vi "Anders_AnalyzeUDP_IRIS_V1_optimized.vi"(10 "Input UDP packet array":i32[][](array[numeric])=array703x1377[968031 elements]) -> (0 "Valid":bool[](array[boolean]), 2 "All good 2":bool, 3 "Return Description":T2(array[cluster]))   [LabVIEW 2018]
panel:
  out "unsigned 8bit integer":u8[](array[numeric])
  in  "Tab Control":T1(tab)
  out "Number of UDP arrays":i32
  out "All good":bool
  out "Ray sequence":u8=12
  out "Returns":u8
  out "Final size":i32=1336
  out "time stamp, ns":u32=459884670
  out "Detector":i32
  out "Line number 2":i32=146
  out "Azimuth(rad)":dbl=0.5140380859375
  out "Elevation(rad)":dbl=-0.232177734375
  out "Checkpoint":bool
  out "Returns OK":bool
  out "RESERVED3=239":bool
  out "Number of rays":u8=53
  out "found rays":i32=53
  out "# completed UDP arrays":i32
  out "size(s)":i32=42322
  # "340-400\n260-280\n97"
  # "1. Wall at 14m\n2. Dual pole= Site A+B crosstalk\n3. Edge spray is range walk"
  # "Analyze UDP IRIS V1"
  # "Ray header (for every ray)"
  # "Returns"
  # "Lidar Packet header"
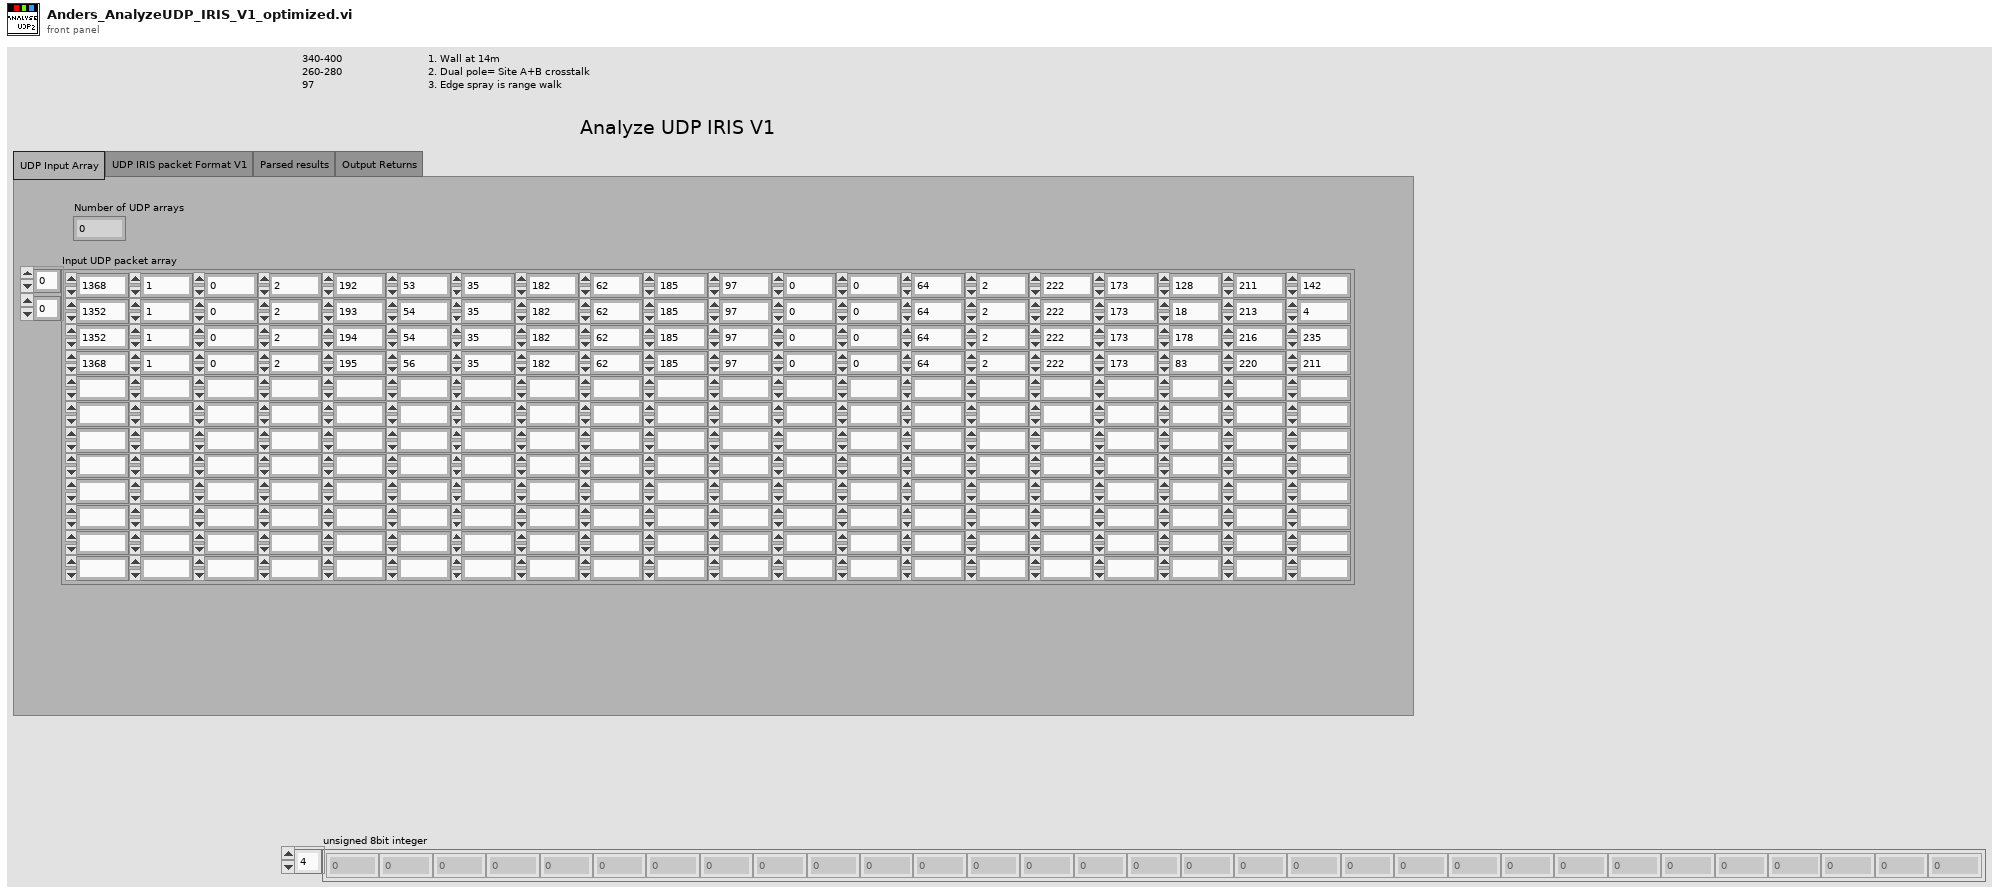
[diagram p1: front panel]
types:
  T1 = enum32{"UDP Input Array", "UDP IRIS packet Format V1", "Parsed results", "Output Returns"}
  T2 = cluster{"Azimuth":dbl, "Elevation":dbl, "Timestamp,ns":u32, "Detector":i32, "Line number":u16, "Range":ext, "Probability":ext, "Reflectance":ext, "Return":ext}[]
  T3 = cluster{dbl, dbl, "u32":u32, i32, u16, ext, ext, ext, i32}
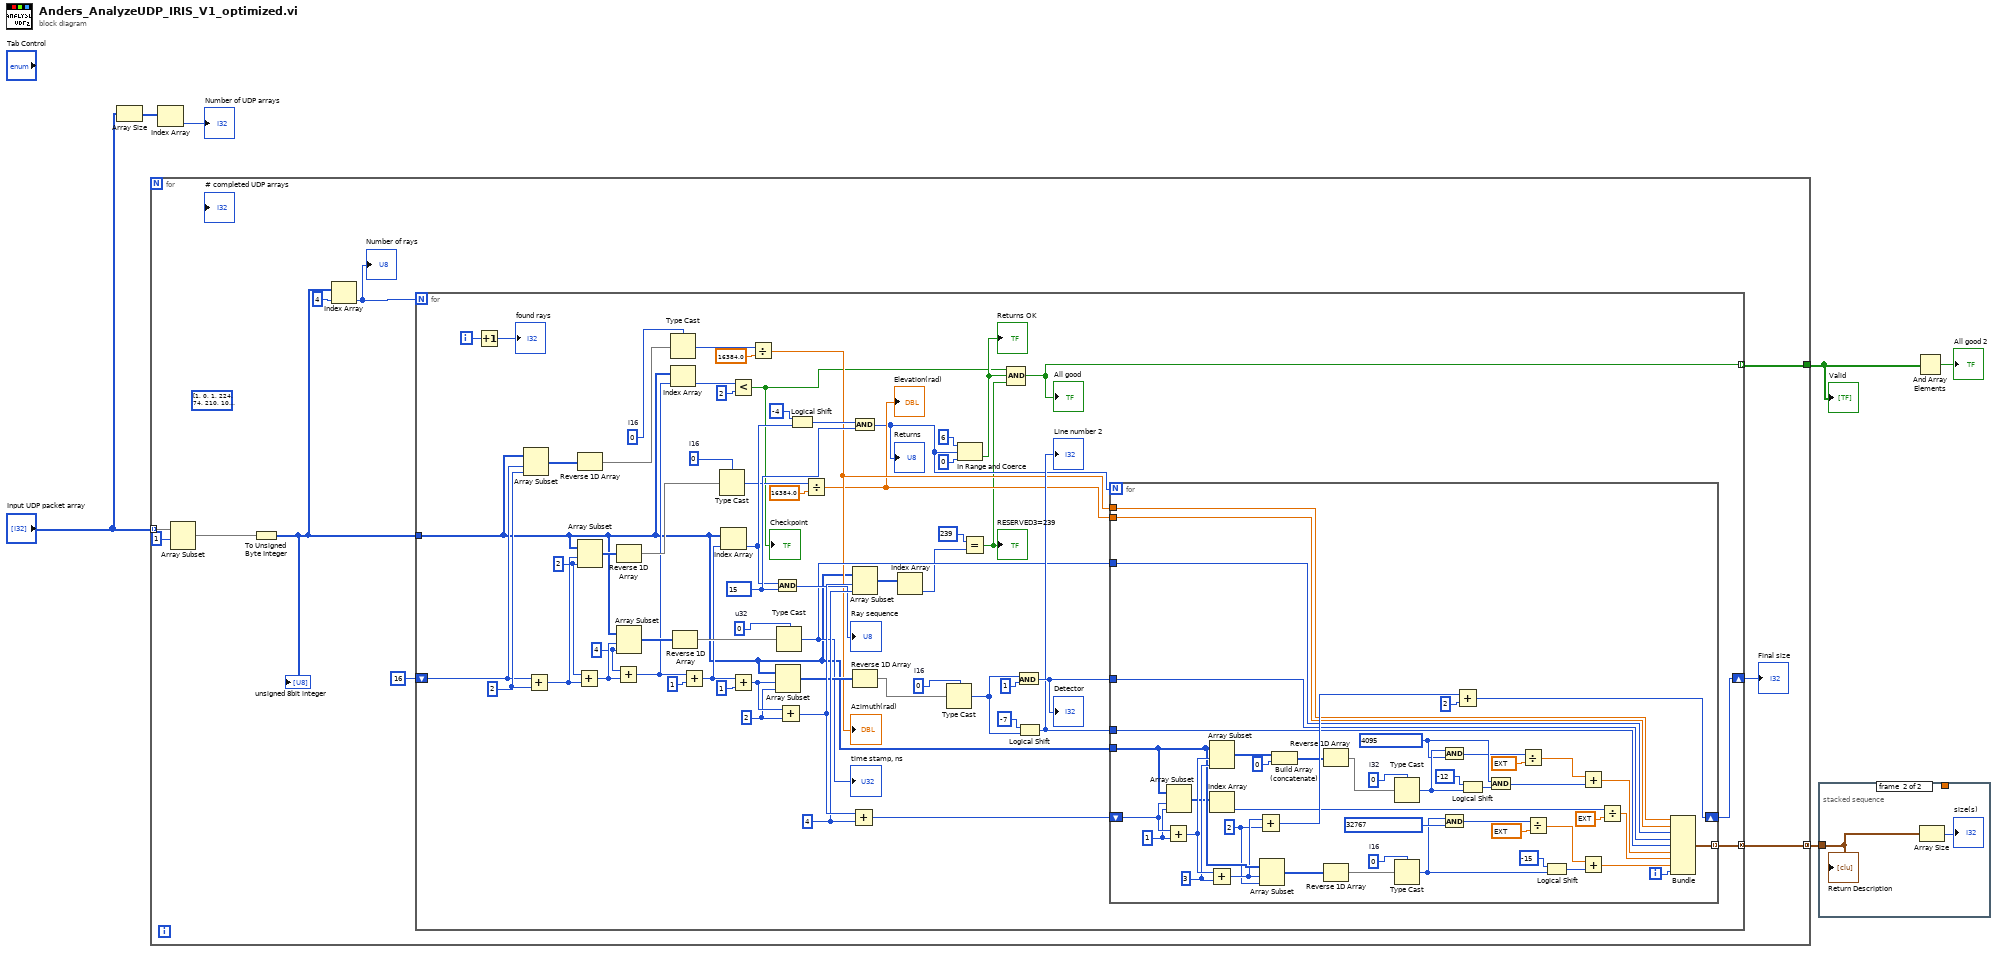
[diagram p0: block diagram]
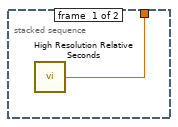
[diagram p2: hidden frame]
diagram:
  n1 = Array Size(array="Input UDP packet array") -> (size(s)=w6:i32[])
  n2 = for {
    tunnel: [w16] -> w3 mode=concatenating
    tunnel: [w15] -> w2
    tunnel: "Input UDP packet array" -> [w14] mode=indexing
    (unwired) u8[] [1, 0, 1, 224, 74, 210, 101, 1, 0, 0, 0, 0, 64, 2, 222, 173, 90, 70, 182, 0, 139, 134, 224, 18, 0, 10, 130, 50, 239, 190, 173, 222, 127, 68, 27, 0, 139, 134, 224, 18, 0, 11, 131, 50, 239, 190, 173, 222, 125, 70, 181, 0, 191, 142, 224, 18, 0, 12, 130, 50, 239, 190, 173, 222, 162, 68, 26, 0, 191, 142, 224, 18, 0, 13, 131, 50, 239, 190, 173, 222, 159, 70, 181, 0, 213, 150, 224, 18, 0, 14, 130, 50, 239, 190, 173, 222, 196, 68, 26, 0, 213, 150, 224, 18, 0, 15, 131, 50, 239, 190, 173, 222, 194, 70, 180, 0, 10, 159, 224, 18, 0, 0, 130, 50, 239, 190, 173, 222, 230, 68, 25, 0, 10, 159, 224, 18, 0, 1, 131, 50, 239, 190, 173, 222, 228, 70, 180, 0, 32, 167, 224, 18, 0, 2, 130, 50, 239, 190, 173, 222, 9, 69, 25, 0, 32, 167, 224, 18, 0, 3, 131, 50, 239, 190, 173, 222, 6, 71, 179, 0, 84, 175, 224, 18, 0, 4, 130, 50, 239, 190, 173, 222, 43, 69, 25, 0, 84, 175, 224, 18, 0, 5, 131, 50, 239, 190, 173, 222, 41, 71, 179, 0, 136, 183, 224, 18, 0, 6, 130, 50, 239, 190, 173, 222, 78, 69, 24, 0, 136, 183, 224, 18, 0, 7, 131, 50, 239, 190, 173, 222, 75, 71, 179, 0, 158, 191, 224, 18, 0, 8, 130, 50, 239, 190, 173, 222, 112, 69, 24, 0, 158, 191, 224, 18, 0, 9, 131, 50, 239, 190, 173, 222, 109, 71, 178, 0, 210, 199, 224, 18, 0, 10, 130, 50, 239, 190, 173, 222, 146, 69, 23, 0, 210, 199, 224, 18, 0, 11, 131, 50, 239, 190, 173, 222, 144, 71, 178, 0, 232, 207, 224, 18, 0, 12, 130, 50, 239, 190, 173, 222, 181, 69, 23, 0, 232, 207, 224, 18, 0, 13, 131, 50, 239, 190, 173, 222, 178, 71, 177, 0, 28, 216, 224, 18, 0, 14, 130, 50, 239, 190, 173, 222, 215, 69, 23, 0, 28, 216, 224, 18, 0, 15, 131, 50, 239, 190, 173, 222, 212, 71, 177, 0, 50, 224, 224, 18, 0, 0, 130, 50, 239, 190, 173, 222, 249, 69, 22, 0, 50, 224, 224, 18, 0, 1, 131, 50, 239, 190, 173, 222, 247, 71, 176, 0, 102, 232, 224, 18, 0, 2, 130, 50, 239, 190, 173, 222, 28, 70, 22, 0, 102, 232, 224, 18, 0, 3, 131, 50, 239, 190, 173, 222, 25, 72, 176, 0, 124, 240, 224, 18, 0, 4, 130, 50, 239, 190, 173, 222, 62, 70, 21, 0, 124, 240, 224, 18, 0, 5, 131, 50, 239, 190, 173, 222, 60, 72, 176, 0, 176, 248, 224, 18, 0, 6, 130, 50, 239, 190, 173, 222, 96, 70, 21, 0, 176, 248, 224, 18, 0, 7, 131, 50, 239, 190, 173, 222, 94, 72, 175, 0, 228, 0, 225, 18, 0, 8, 130, 50, 239, 190, 173, 222, 131, 70, 20, 0, 228, 0, 225, 18, 0, 9, 131, 50, 239, 190, 173, 222, 128, 72, 175, 0, 251, 8, 225, 18, 0, 10, 130, 50, 239, 190, 173, 222, 165, 70, 20, 0, 251, 8, 225, 18, 0, 11, 131, 50, 239, 190, 173, 222, 163, 72, 174, 0, 47, 17, 225, 18, 0, 12, 130, 50, 239, 190, 173, 222, 200, 70, 20, 0, 47, 17, 225, 18, 0, 13, 131, 50, 239, 190, 173, 222, 197, 72, 174, 0, 69, 25, 225, 18, 0, 14, 130, 50, 239, 190, 173, 222, 234, 70, 19, 0, 69, 25, 225, 18, 0, 15, 131, 50, 239, 190, 173, 222, 232, 72, 174, 0, 121, 33, 225, 18, 0, 0, 130, 50, 239, 190, 173, 222, 12, 71, 19, 0, 121, 33, 225, 18, 0, 1, 131, 50, 239, 190, 173, 222, 10, 73, 173, 0, 143, 41, 225, 18, 0, 2, 130, 50, 239, 190, 173, 222, 47, 71, 18, 0, 143, 41, 225, 18, 0, 3, 131, 50, 239, 190, 173, 222, 44, 73, 173, 0, 195, 49, 225, 18, 0, 4, 130, 50, 239, 190, 173, 222, 81, 71, 18, 0, 195, 49, 225, 18, 0, 5, 131, 50, 239, 190, 173, 222, 79, 73, 172, 0, 217, 57, 225, 18, 0, 6, 130, 50, 239, 190, 173, 222, 116, 71, 18, 0, 217, 57, 225, 18, 0, 7, 131, 50, 239, 190, 173, 222, 113, 73, 172, 0, 13, 66, 225, 18, 0, 8, 130, 50, 239, 190, 173, 222, 150, 71, 17, 0, 13, 66, 225, 18, 0, 9, 131, 50, 239, 190, 173, 222, 10, 193, 204, 0, 249, 138, 240, 18, 0, 10, 4, 51, 239, 190, 173, 222, 47, 191, 38, 0, 249, 138, 240, 18, 0, 11, 5, 51, 239, 190, 173, 222, 45, 193, 204, 0, 15, 147, 240, 18, 0, 12, 4, 51, 239, 190, 173, 222, 82, 191, 38, 0, 15, 147, 240, 18, 0, 29, 5, 51, 239, 190, 173, 222, 63, 48, 0, 0, 96, 35, 8, 0, 79, 193, 205, 0, 67, 155, 240, 18, 0, 14, 4, 51, 239, 190, 173, 222, 116, 191, 39, 0, 67, 155, 240, 18, 0, 31, 5, 51, 239, 190, 173, 222, 63, 192, 0, 0, 184, 35, 8, 0, 114, 193, 205, 0, 119, 163, 240, 18, 0, 0, 4, 51, 239, 190, 173, 222, 150, 191, 39, 0, 119, 163, 240, 18, 0, 1, 5, 51, 239, 190, 173, 222, 148, 193, 205, 0, 141, 171, 240, 18, 0, 2, 4, 51, 239, 190, 173, 222, 185, 191, 39, 0, 141, 171, 240, 18, 0, 19, 5, 51, 239, 190, 173, 222, 63, 48, 0, 0, 8, 34, 8, 0, 182, 193, 206, 0, 194, 179, 240, 18, 0, 20, 4, 51, 239, 190, 173, 222, 255, 140, 24, 0, 160, 13, 0, 0, 219, 191, 40, 0, 194, 179, 240, 18, 0, 5, 5, 51, 239, 190, 173, 222, 217, 193, 206, 0, 216, 187, 240, 18, 0, 6, 4, 51, 239, 190, 173, 222, 254, 191, 40, 0, 216, 187, 240, 18, 0, 23, 5, 51, 239, 190, 173, 222, 63, 192, 0, 0, 224, 40, 8, 0, 251, 193, 207, 0, 12, 196, 240, 18, 0, 8, 4, 51, 239, 190, 173, 222, 32, 192, 41, 0, 12, 196, 240, 18, 0, 25, 5, 51, 239, 190, 173, 222, 63, 192, 0, 0, 32, 37, 8, 0, 29, 194, 207, 0, 34, 204, 240, 18, 0, 26, 4, 51, 239, 190, 173, 222, 255, 11, 26, 0, 160, 5, 0, 0, 66, 192, 41, 0, 34, 204, 240, 18, 0, 27, 5, 51, 239, 190, 173, 222, 63, 192, 0, 0, 104, 37, 8, 0, 64, 194, 207, 0, 86, 212, 240, 18, 0, 28, 4, 51, 239, 190, 173, 222, 255, 251, 26, 0, 224, 2, 0, 0, 101, 192, 41, 0, 86, 212, 240, 18, 0, 29, 5, 51, 239, 190, 173, 222, 63, 192, 0, 0, 136, 40, 8, 0, 98, 194, 208, 0, 108, 220, 240, 18, 0, 30, 4, 51, 239, 190, 173, 222, 255, 11, 26, 0, 144, 4, 0, 0, 135, 192, 42, 0, 108, 220, 240, 18, 0, 31, 5, 51, 239, 190, 173, 222, 63, 192, 0, 0, 168, 36, 8, 0, 132, 194, 208, 0, 160, 228, 240, 18, 0, 16, 4, 51, 239, 190, 173, 222, 255, 219, 25, 0, 168, 5, 0, 0, 169, 192, 42, 0, 160, 228, 240, 18, 0, 17, 5, 51, 239, 190, 173, 222, 63, 48, 0, 0, 72, 38, 8, 0, 167, 194, 208, 0, 212, 236, 240, 18, 0, 18, 4, 51, 239, 190, 173, 222, 255, 140, 24, 0, 168, 10, 0, 0, 204, 192, 43, 0, 212, 236, 240, 18, 0, 19, 5, 51, 239, 190, 173, 222, 63, 192, 0, 0, 0, 42, 8, 0, 0, 7, 131, 50, 239, 190, 173, 222, 63, 95, 3, 0, 88, 92, 8, 0, 255, 28, 22, 0, 24, 3, 0, 0, 0, 0, 0, 0, 0, 0, 0, 0, 0, 0, 0, 0, 0, 0, 0, 0, 0, 0, 0, 0, 0, 0, 0, 0] ("subarray")
    n3 = Array Subset(array=w14, index=1) -> (w13:i32[])  [unwired: 1 in]
    n4 = To Unsigned Byte Integer(number=w13) -> (unsigned 8bit integer=w7:u8[])
    "unsigned 8bit integer" <- w7
    n5 = Index Array(array=w7, index=4) -> (element=w8:u8)
    "Number of rays" <- w8
    n6 = for {
      N: w8 -> [_]
      tunnel: w7 -> [w19]
      shift-right: [w61] -> w12
      shift-left: 16 -> [w58]
      tunnel: [w18] -> w15 mode=indexing
      tunnel: [w17] -> w16 mode=concatenating
      i -> [w26]
      w47 = u16 0  # i16
      w50 = i16 0  # i16
      w51 = i16 0  # i16
      w56 = u32 0  # u32
      w64 = u16 15 ("Mask")
      w67 = 4 ("length")
      w69 = 2 ("length")
      w74 = 4 ("length")
      w72 = 2 ("length")
      w71 = 2 ("length")
      n7 = Increment(x=w26) -> (x+1=→"found rays":i32)
      n8 = Array Subset(array=w19, index=w58, length=w71) -> (w53:u8[])
      n9 = Add(x=w58, y=w71) -> (x+y=w73:i32)
      n10 = Add(x=w72, y=w73) -> (x+y=w75:i32)
      n11 = Reverse 1D Array(array=w53) -> (reversed array=w52:u8[])
      n12 = Array Subset(array=w19, index=w73, length=w72) -> (w49:u8[])
      n13 = Add(x=w74, y=w75) -> (x+y=w22:i32)
      n14 = Reverse 1D Array(array=w49) -> (reversed array=w42:u8[])
      n15 = Array Subset(array=w19, index=w75, length=w74) -> (w55:u8[])
      n16 = Type Cast(type=w51, x=w52) -> (*(type *) &x=w38:i16)
      n17 = Index Array(array=w19, index=w22) -> (element=w21:u8)
      n18 = Reverse 1D Array(array=w55) -> (reversed array=w54:u8[])
      n19 = Add(x=w22, y=1 ("length")) -> (x+y=w20:i32)
      n20 = Type Cast(type=w50, x=w42) -> (*(type *) &x=w40:i16)
      n21 = Index Array(array=w19, index=w20) -> (element=w63:u8)
      n22 = Less?(x=w21, y=u8 2) -> (x < y?=w23:bool)
      "Checkpoint" <- w23
      n23 = Add(x=w20, y=1 ("length")) -> (x+y=w70:i32)
      n24 = Divide(x=w38, y=16384.0 ("x*2^n")) -> (x/y=w34:dbl)
      "Azimuth(rad)" <- w34
      n25 = And(x=w63, y=w64) -> (x .and. y?=→"Ray sequence":u16)
      n26 = Array Subset(array=w19, index=w70, length=w69) -> (w48:u8[])
      n27 = Type Cast(type=w56, x=w54) -> (*(type *) &x=w35:u32)
      "time stamp, ns" <- w35
      n28 = Add(x=w70, y=w69) -> (x+y=w68:i32)
      n29 = Logical Shift(y=i16 -4, x=w63) -> (x << y=w65:u8)
      n30 = Divide(x=w40, y=16384.0 ("x*2^n")) -> (x/y=w33:dbl)
      "Elevation(rad)" <- w33
      n31 = Add(x=w68, y=w67) -> (x+y=w66:i32)
      n32 = And(x=w65, y=w64) -> (x .and. y?=w32:u16)
      "Returns" <- w32
      n33 = Array Subset(array=w19, index=w68, length=w67) -> (w30:u8[])
      n34 = Reverse 1D Array(array=w48) -> (reversed array=w46:u8[])
      n35 = Index Array(array=w30) -> (element=w29:u8)  [unwired: 1 in]
      n36 = Type Cast(type=w47, x=w46) -> (*(type *) &x=w43:u16)
      n37 = In Range and Coerce(upper limit=u16 6, x=w32, lower limit=u16 0) -> (In Range?=w28:bool)  [unwired: 1 out]
      "Returns OK" <- w28
      n38 = Equal?(x=u8 239, y=w29) -> (x = y?=w27:bool)
      "RESERVED3=239" <- w27
      n39 = Compound Arithmetic op=AND(w23, w28, w27) -> (w18:bool)
      "All good" <- w18
      n40 = And(x=w43, y=1 ("Mask")) -> (x .and. y?=w37:i32)
      "Detector" <- w37
      n41 = Logical Shift(y=i16 -7, x=w43) -> (x << y=w36:u16)
      "Line number 2" <- w36
      n42 = for {
        N: w32 -> [_]
        tunnel: w19 -> [w119]
        shift-right: [w115] -> w61
        shift-left: w66 -> [w123]
        tunnel: w34 -> [w87]
        tunnel: w33 -> [w86]
        tunnel: w35 -> [w85]
        tunnel: w37 -> [w84]
        tunnel: w36 -> [w83]
        tunnel: [w78] -> w17 mode=indexing
        i -> [w81]
        w109 = 4095 ("Mask")
        w112 = i16 0  # i16
        w113 = 0  # i32
        w117 = 2 ("length")
        w120 = 3 ("length")
        w122 = 1 ("length")
        n43 = Add(x=w123, y=w122) -> (x+y=w121:i32)
        n44 = Array Subset(array=w119, index=w123, length=w122) -> (w114:u8[])
        n45 = Add(x=w121, y=w120) -> (x+y=w118:i32)
        n46 = Array Subset(array=w119, index=w121, length=w120) -> (w101:u8[])
        n47 = Index Array(array=w114) -> (element=w90:u8)  [unwired: 1 in]
        n48 = Add(x=w118, y=w117) -> (x+y=w116:i32)
        n49 = Array Subset(array=w119, index=w118, length=w117) -> (w99:u8[])
        n50 = Build Array (concatenate)(w101, u8 0) -> (w102:u8[])
        n51 = Reverse 1D Array(array=w102) -> (reversed array=w100:u8[])
        n52 = Reverse 1D Array(array=w99) -> (reversed array=w98:u8[])
        n53 = Type Cast(type=w113, x=w100) -> (*(type *) &x=w110:i32)
        n54 = Type Cast(type=w112, x=w98) -> (*(type *) &x=w96:i16)
        n55 = And(x=w110, y=w109) -> (x .and. y?=w106:i32)
        n56 = And(x=w96, y=32767 ("Mask")) -> (x .and. y?=w93:i32)
        n57 = Add(x=w116, y=2 ("length")) -> (x+y=w115:i32)
        n58 = Logical Shift(y=i16 -12, x=w110) -> (x << y=w108:i32)
        n59 = And(x=w109, y=w108) -> (x .and. y?=w104:i32)
        n60 = Divide(x=w106, y=ext 4096.0 ("x*2^n")) -> (x/y=w105:ext)
        n61 = Divide(x=w93, y=ext 32768.0 ("x*2^n")) -> (x/y=w91:ext)
        n62 = Logical Shift(y=i16 -15, x=w96) -> (x << y=w94:i16)
        n63 = Add(x=w105, y=w104) -> (x+y=w79:ext)
        n64 = Add(x=w91, y=w94) -> (x+y=w80:ext)
        n65 = Divide(x=w90, y=ext 255.0 ("x*2^n")) -> (x/y=w82:ext)
        n66 = Bundle(w87, w86, "u32"=w85, w84, w83, w79, w82, w80, w81) -> (w78:T3)  [unwired: 1 in]
      }
    }
    "Final size" <- w12
  }
  "Valid" <- w2
  n67 = Index Array(array=w6) -> (element=→"Number of UDP arrays":i32)  [unwired: 1 in]
  n68 = stacked-sequence {
    tunnel: w3 -> [_ w125]
    tunnel: [w124 _] -> _
    frame #0 {
      n69 = call <vilib>:"High Resolution Relative Seconds.vi"() -> ("relative seconds"=w124:dbl)
    }
    frame #1 {
      n70 = Array Size(array=w125) -> (size(s)=→"size(s)":i32)
      "Return Description" <- w125
    }
  }
  n71 = And Array Elements(Boolean array=w2) -> (logical AND=→"All good 2":bool)
